vi "Wait_Seconds_with_display.vi"(2 "Message":string, 3 "Seconds to wait":dbl=1.0 format="%.2f") -> (1 "Stopped":bool)   [LabVIEW 2011]
doc: "Waits the number of seconds specified by the Seconds to Wait input, divided by the time dilation factor, if used."
uses:
  Globals/Meas_global.vi
panel:
  in  "stop":bool
  out "Seconds waited":u32(slide) scale=0.0..900.0
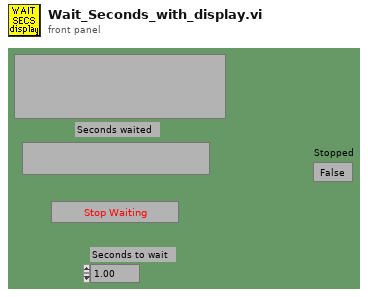
[diagram p1: front panel]
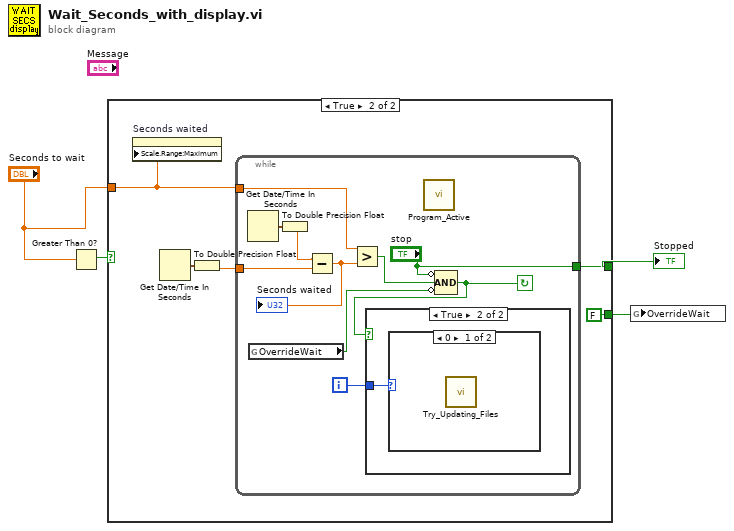
[diagram p0: block diagram]
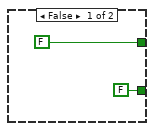
[diagram p2: hidden frame]
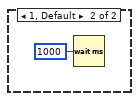
[diagram p4: hidden frame]
diagram:
  n1 = Greater Than 0?(x="Seconds to wait") -> (x > 0?=w3:bool)
  n2 = case shown="True" w3 {
    tunnel: [FALSE ("stop") w11] -> w4
    tunnel: "Seconds to wait" -> [_ w9]
    tunnel: [FALSE FALSE] -> w1
    frame False {
    }
    frame True {
      n3 = property on="Seconds waited" class="Slide (strict)"("Scale.Range:Maximum"=w9) -> ()  [unwired: 2 in, 2 out]
      n4 = Get Date/Time In Seconds() -> (seconds since 1Jan1904=w8:timestamp)
      n5 = To Double Precision Float(number=w8) -> (double precision float=w10:dbl)
      n6 = while {
        tunnel: ["stop"] -> w11
        tunnel: w9 -> [w18]
        tunnel: w10 -> [w21]
        i -> [w13]
        stop <- w14 continue-if-true
        n7 = Get Date/Time In Seconds() -> (seconds since 1Jan1904=w15:timestamp)
        n8 = global read "Meas_global.vi" "OverrideWait"() -> (w12:bool)
        n9 = To Double Precision Float(number=w15) -> (double precision float=w16:dbl)
        n10 = Subtract(x=w16, y=w21) -> (x-y=w17:dbl)
        "Seconds waited" <- w17
        n11 = Greater?(x=w18, y=w17) -> (0:w20:bool)
        n12 = call "Program_Active.vi"() -> ()  [unwired: 1 in]
        n13 = Compound Arithmetic op=AND(invert "stop", w20, invert w12) -> (w14:bool)
        n14 = case shown="True" w14 {
          tunnel: w13 -> [_ w22]
          frame False {
          }
          frame True {
            n15 = case shown="0" w22 {
              frame 0 {
                n16 = call "Try_Updating_Files.vi"() -> ()  [unwired: 4 out]
              }
              frame 1, Default {
                n17 = Wait (ms)(milliseconds to wait=u32 1000) -> ()  [unwired: 1 out]
              }
            }
          }
        }
      }
    }
  }
  "Stopped" <- w4
  n18 = global write "Meas_global.vi" "OverrideWait"(w1) -> ()
